vi "LaserCal-Process Data (PT).vi"(7 "Power (W)":dbl, 9 "I-O Data in":T1, 11 "error in (no error)":errorcluster, 12 "Seq Index":T2) -> (10 "I-O Data out":T1, 15 "error out":errorcluster)   [LabVIEW 2015]
uses:
  Typedefs/LaserCal-StimConList Element.ctl
  Typedefs/LaserCal-Data (PT).ctl
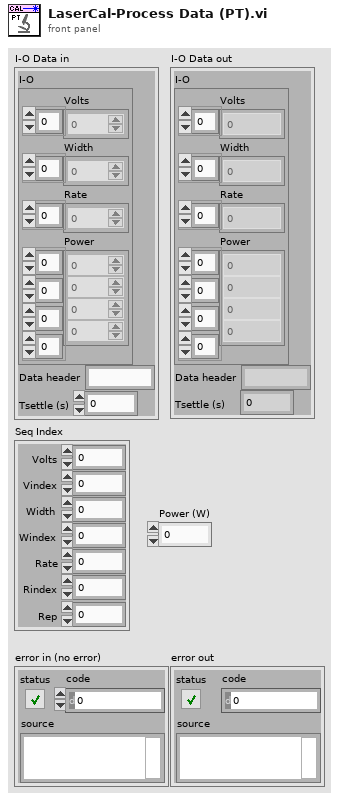
[diagram p1: front panel]
types:
  T1 = typedef "LaserCal-Data (PT).ctl" = cluster{"I-O":cluster{"Volts":dbl[], "Width":dbl[], "Rate":dbl[], "Power":dbl[][][][]}, "Data header":string, "Tsettle (s)":dbl}
  T2 = typedef "LaserCal-StimConList Element.ctl" = cluster{"Volts":dbl, "Vindex":i32, "Width":dbl, "Windex":i32, "Rate":dbl, "Rindex":i32, "Rep":i32}
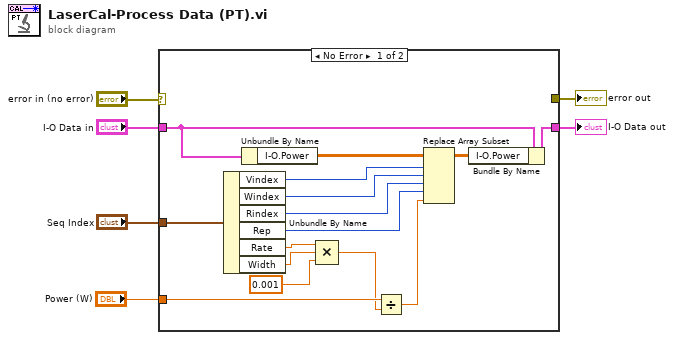
[diagram p0: block diagram]
diagram:
  n1 = case shown="No Error" "error in (no error)" {
    selector: "error in (no error)" -> [_ w23]
    tunnel: [_ w23] -> w2
    tunnel: "I-O Data in" -> [w21 w22]
    tunnel: [w20 w22] -> w4
    tunnel: "Seq Index" -> [w17 _]
    tunnel: "Power (W)" -> [w12 _]
    frame No Error {
      n2 = Unbundle By Name(w17) -> ("Vindex"=w16:i32, "Windex"=w15:i32, "Rindex"=w14:i32, "Rep"=w13:i32, "Rate"=w10:dbl, "Width"=w9:dbl)
      n3 = Unbundle By Name(w21) -> ("I-O.Power"=w19:dbl[][][][])
      n4 = Compound Arithmetic op=MULTIPLY(w10, w9, 0.001) -> (w7:dbl)
      n5 = Divide(x=w12, y=w7) -> (x/y=w11:dbl)
      n6 = Replace Array Subset(array=w19, new element=w11, index (dim 0)=w16, index (dim 1)=w15, index (dim 2)=w14, index (dim 3)=w13) -> (w18:dbl[][][][])
      n7 = Bundle By Name(cluster=w21, "I-O.Power"=w18) -> (w20:T1)
    }
    frame Error {
    }
  }
  "I-O Data out" <- w4
  "error out" <- w2
